vi "fmt_convertChannelIndexToColumnIndex.vi"(9 "TimeColumnMode":T1, 10 "channel index":i32) -> (1 "time column index":i32, 2 "data column index":i32)   [LabVIEW 2017, in "NI_ExcelFile.lvlib"]
uses:
  <vilib>/express/express shared/NI_ExcelFile/NI_ExcelFile.lvlib
  <vilib>/express/express shared/NI_ExcelFile/Ctrls/TimeColumnMode.ctl
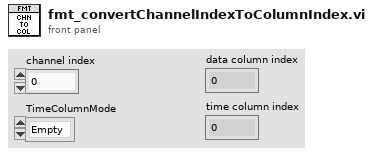
[diagram p1: front panel]
types:
  T1 = typedef "NI_ExcelFile.lvlib/TimeColumnMode.ctl" = enum16{"Empty", "OnePerCh", "One"}
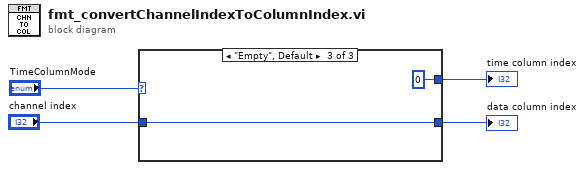
[diagram p0: block diagram]
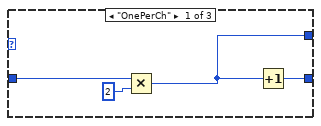
[diagram p2: hidden frame]
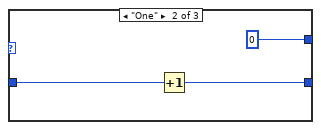
[diagram p3: hidden frame]
diagram:
  n1 = case shown="\"Empty\", Default" "TimeColumnMode" {
    tunnel: "channel index" -> [w8 w11 w13]
    tunnel: [w6 w10 w13] -> w2
    tunnel: [w5 0 ("channel index") 0 ("channel index")] -> w1
    frame "OnePerCh" {
      n2 = Multiply(x=w8, y=2) -> (x*y=w5:i32)
      n3 = Increment(x=w5) -> (x+1=w6:i32)
    }
    frame "One" {
      n4 = Increment(x=w11) -> (x+1=w10:i32)
    }
    frame "Empty", Default {
    }
  }
  "data column index" <- w2
  "time column index" <- w1
